vi "niFpgaBuild_Global_ParameterTags.vi"() -> ()   [LabVIEW 2017]
panel:
  out "ViToVhdlMapText":string="timingViolationPostMungingViToVhdlMap.txt"
  out "ActiveJobList":path=path "rvi/CDR/niFpgaActiveJobList.json"
  out "RegisterMap":string="RegisterMap.dat"
  out "SimulationResults":string="SimulationResults.lvtxt"
  out "CodeGenerationResults":string="CodeGenerationResults.lvtxt"
  out "BuildResults":string="BuildResults.lvtxt"
  out "BuildInformation":string="BuildInformation.lvtxt"
  out "CompileStatusFilename":string="CompileStatus.lvtxt"
  out "BuildInstructions":string="BuildInstructions.lvtxt"
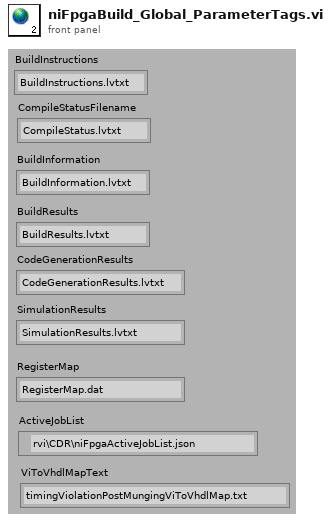
[diagram p1: front panel]
diagram:
